vi "HAPS_MCU_Element_CMD.vi"(5 "set_ele":T3, 7 "HAPS_MCU_ELE_Func.":T2, 8 "error in":errorcluster, 11 "Function":T1={"Tx/Rx"=enum."Rx", "Enable?"=enum."On", "Source"=enum."MCU"}) -> (0 "error out":errorcluster, 3 "Data":string)   [LabVIEW 2023, in "HAPS.lvlib"]
uses:
  HAPS.lvlib
  HAPS_MCU_ELE_Func.ctl
  set_ele.ctl
  MCU_Function.ctl
panel:
  out "Time(ms)":dbl
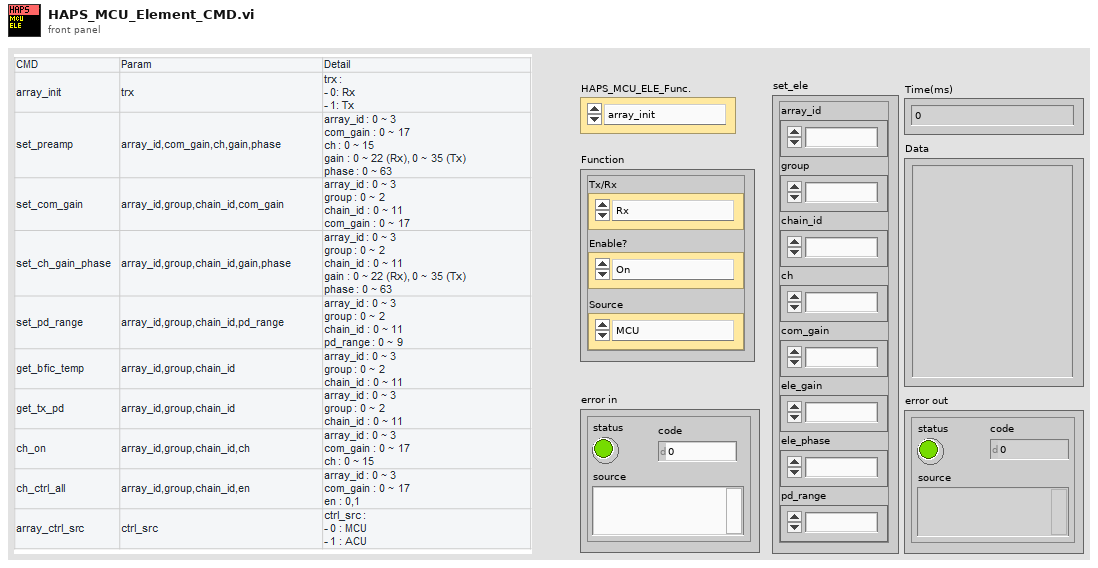
[diagram p1: front panel]
types:
  T1 = typedef "HAPS.lvlib/MCU_Function.ctl" = cluster{"Tx/Rx":enum16{"Rx", "Tx"}, "Enable?":enum16{"OFF", "On"}, "Source":enum16{"MCU", "ACU"}}
  T2 = typedef "HAPS.lvlib/HAPS_MCU_ELE_Func.ctl" = enum16{"array_init", "set_com_gain", "set_ch_gain_phase", "set_pd_range", "get_preamp_temp", "get_bfic_temp", "get_tx_pd", "ch_on", "ch_on_2", "ch_ctrl_all", "array_ctrl_src"}
  T3 = typedef "HAPS.lvlib/set_ele.ctl" = cluster{"ch":i32, "chain_id":i32, "group":i32, "array_id":i32, "ele_phase":i32, "ele_gain":i32, "com_gain":i32, "pd_range":i32}
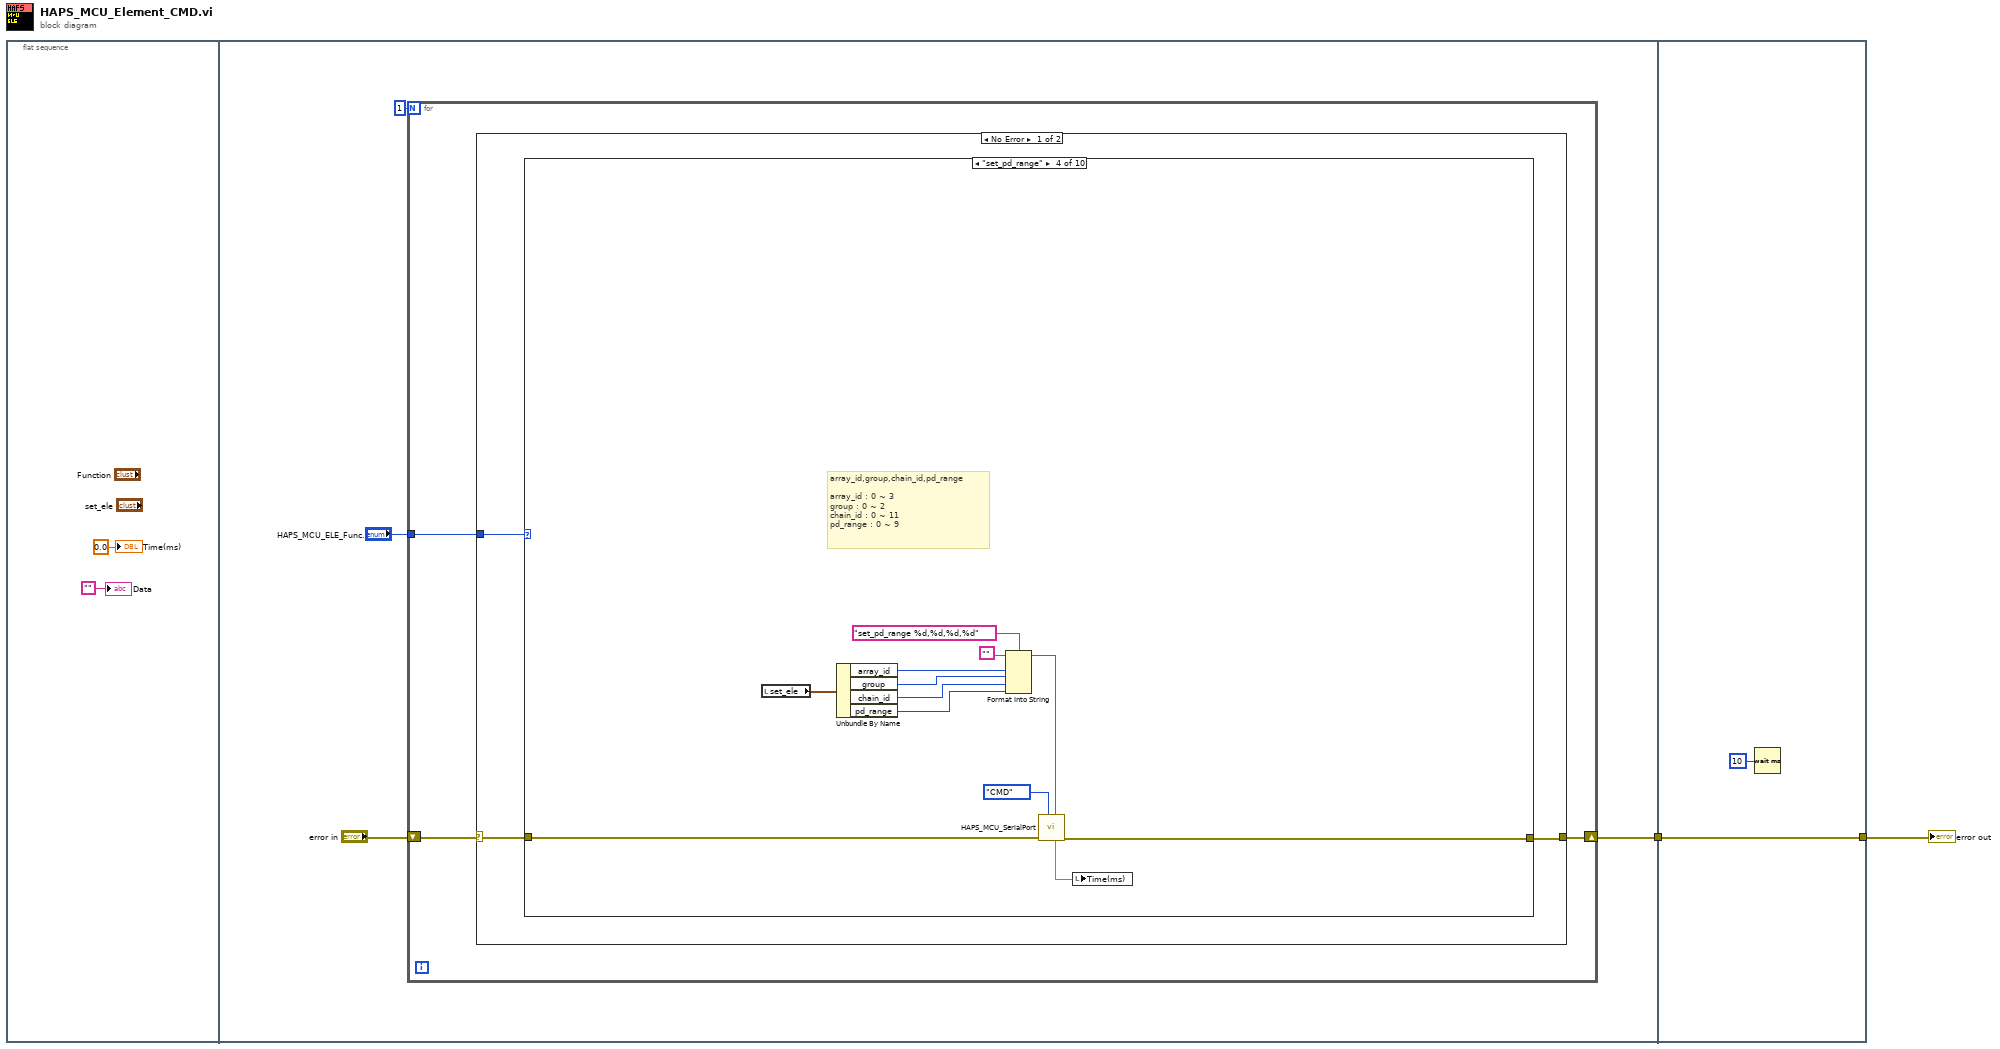
[diagram p0: block diagram]
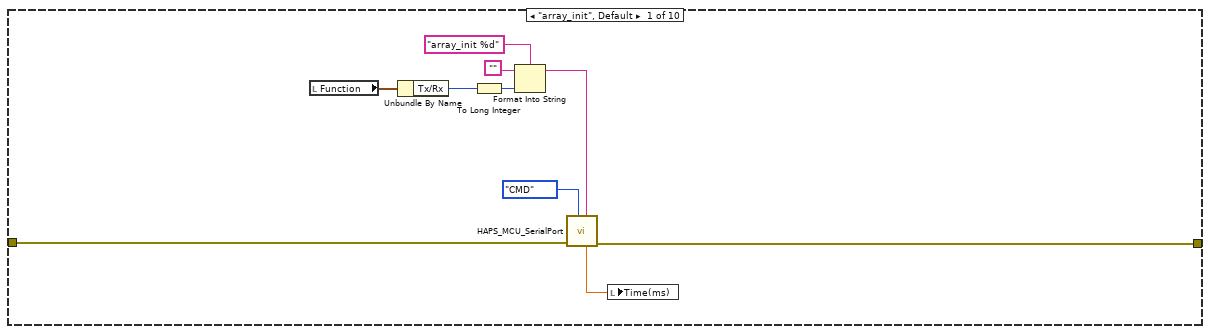
[diagram p2: hidden frame]
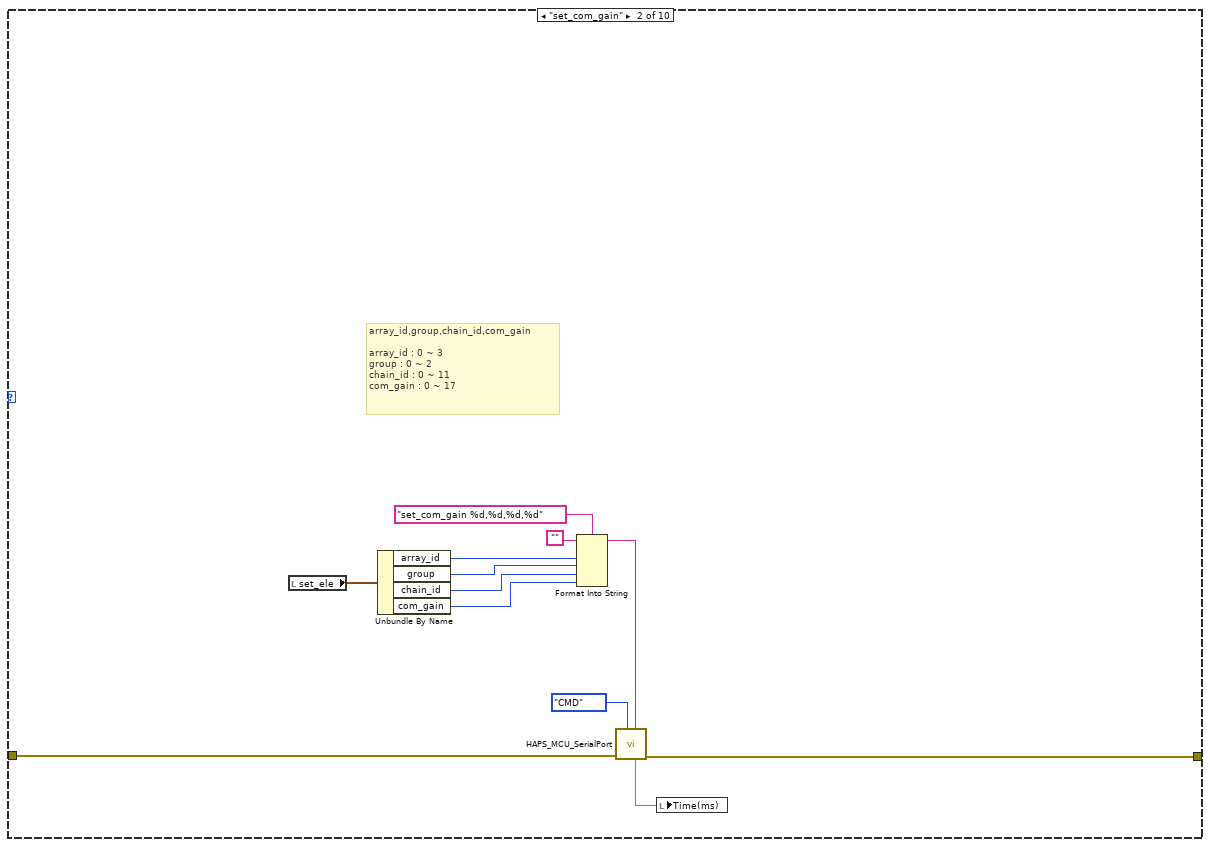
[diagram p3: hidden frame]
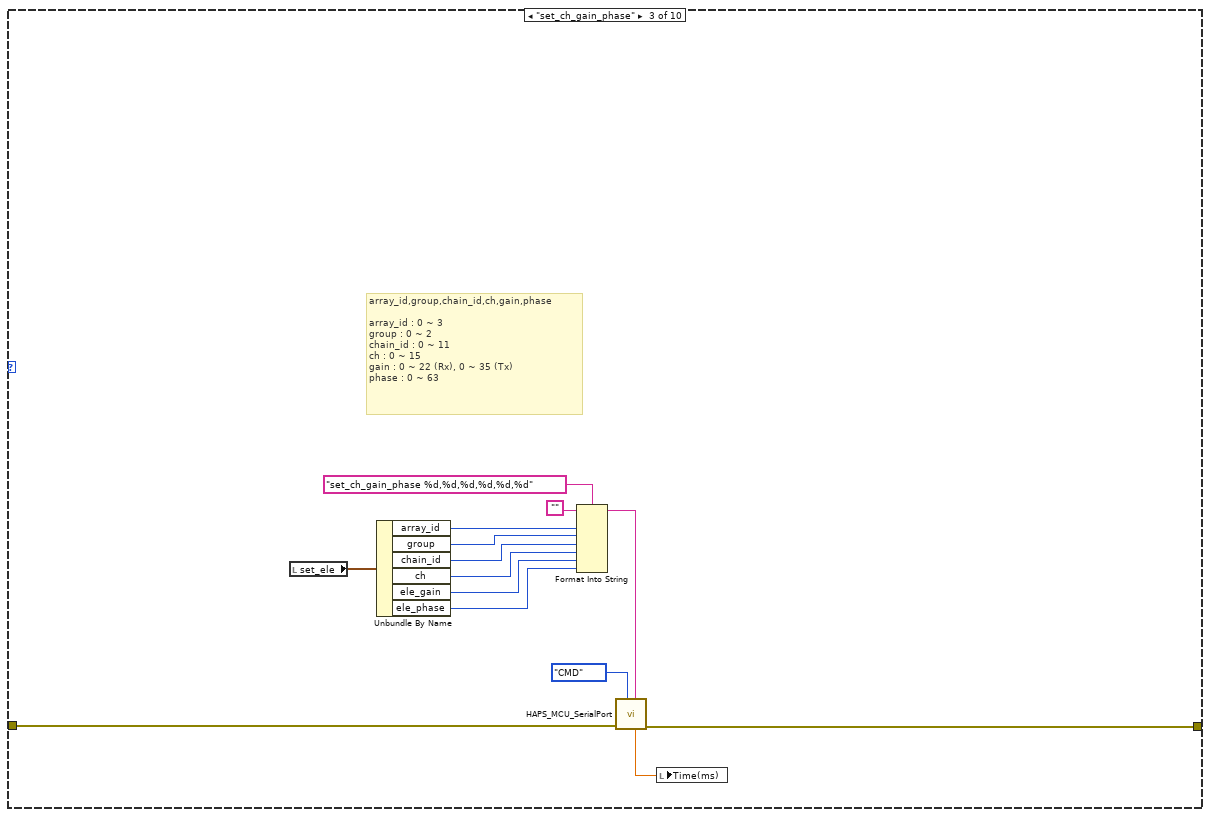
[diagram p4: hidden frame]
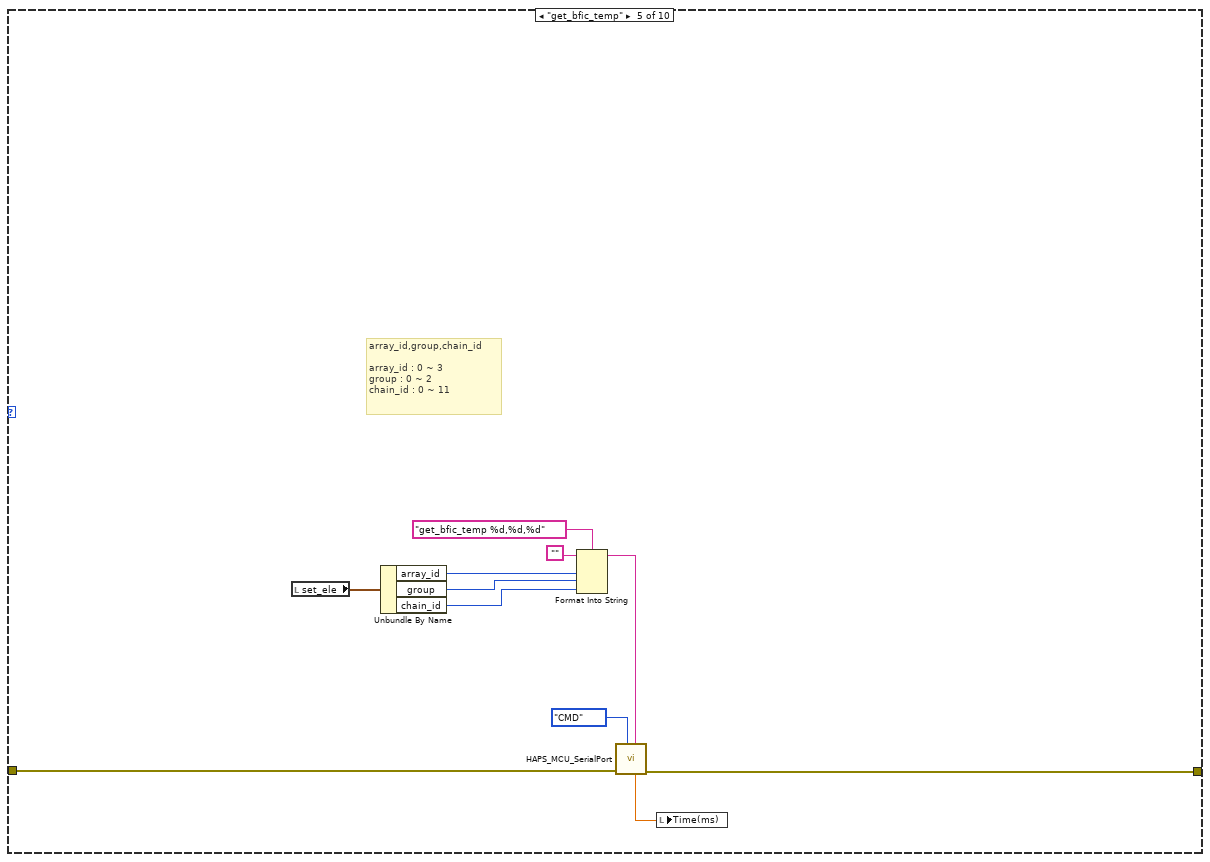
[diagram p5: hidden frame]
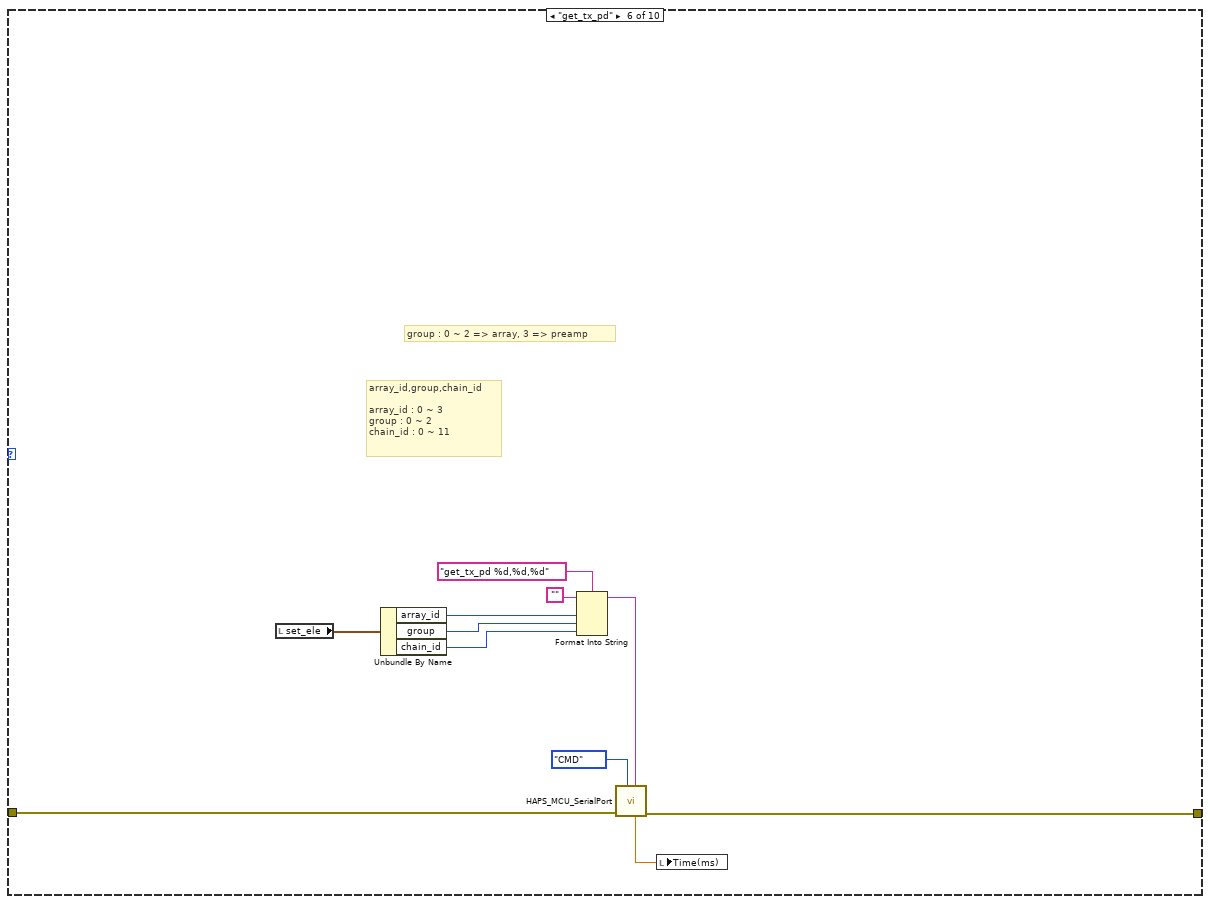
[diagram p6: hidden frame]
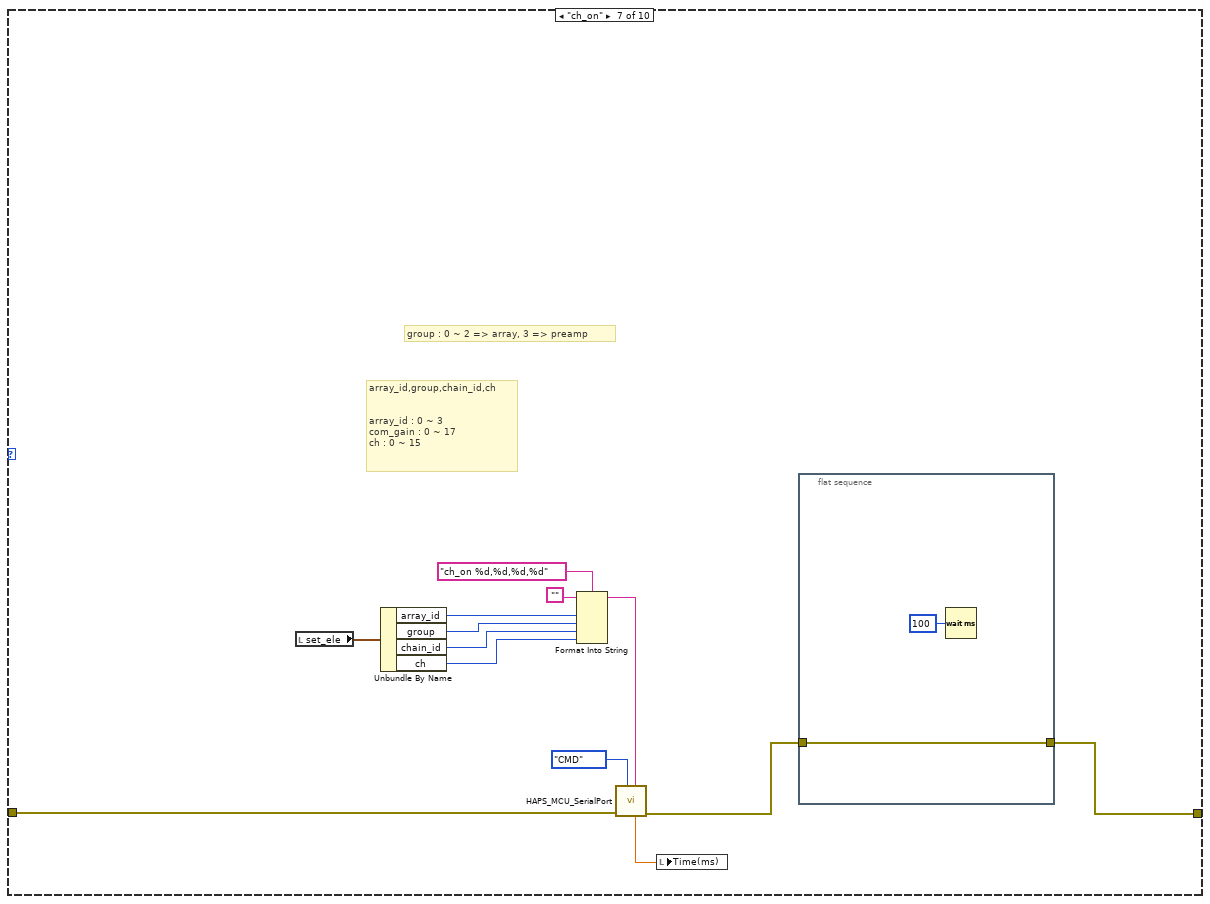
[diagram p7: hidden frame]
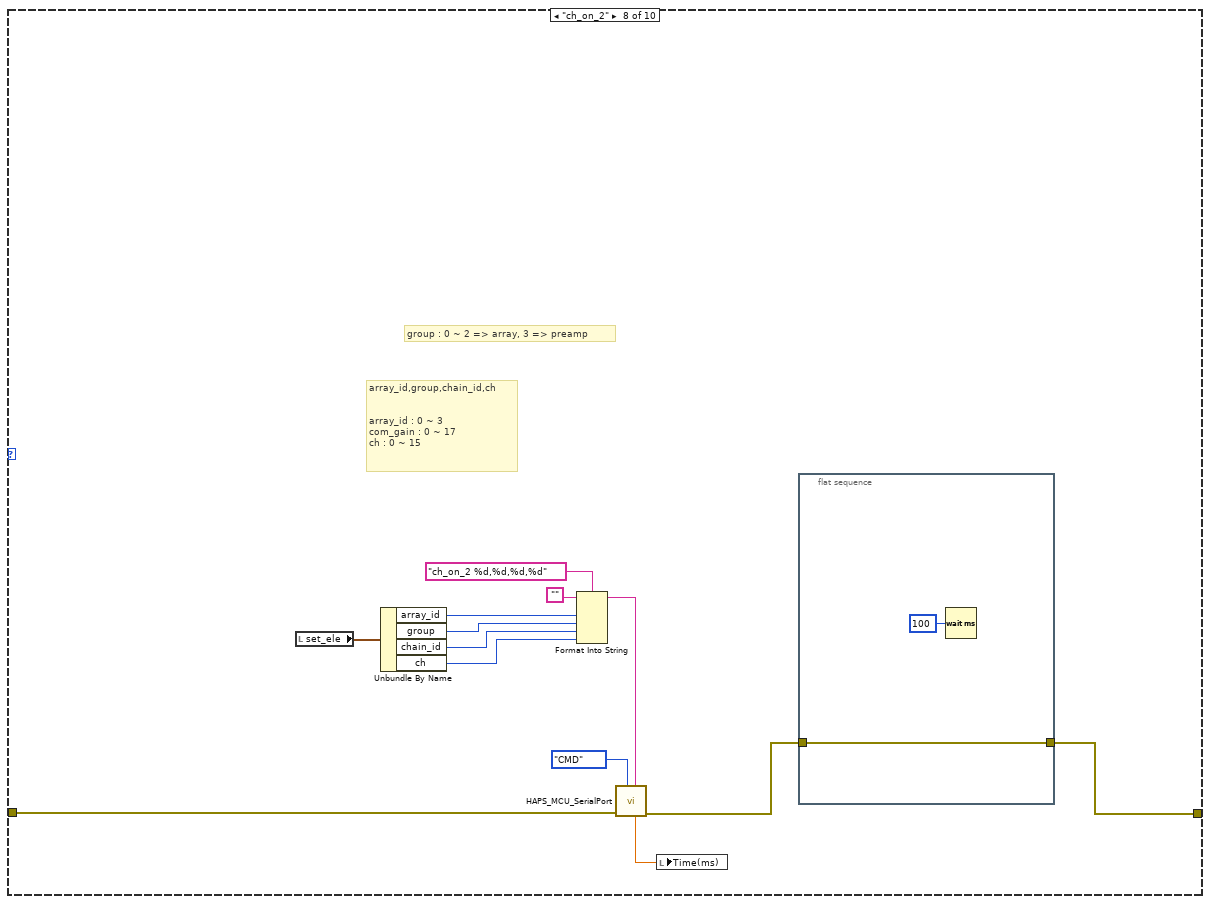
[diagram p8: hidden frame]
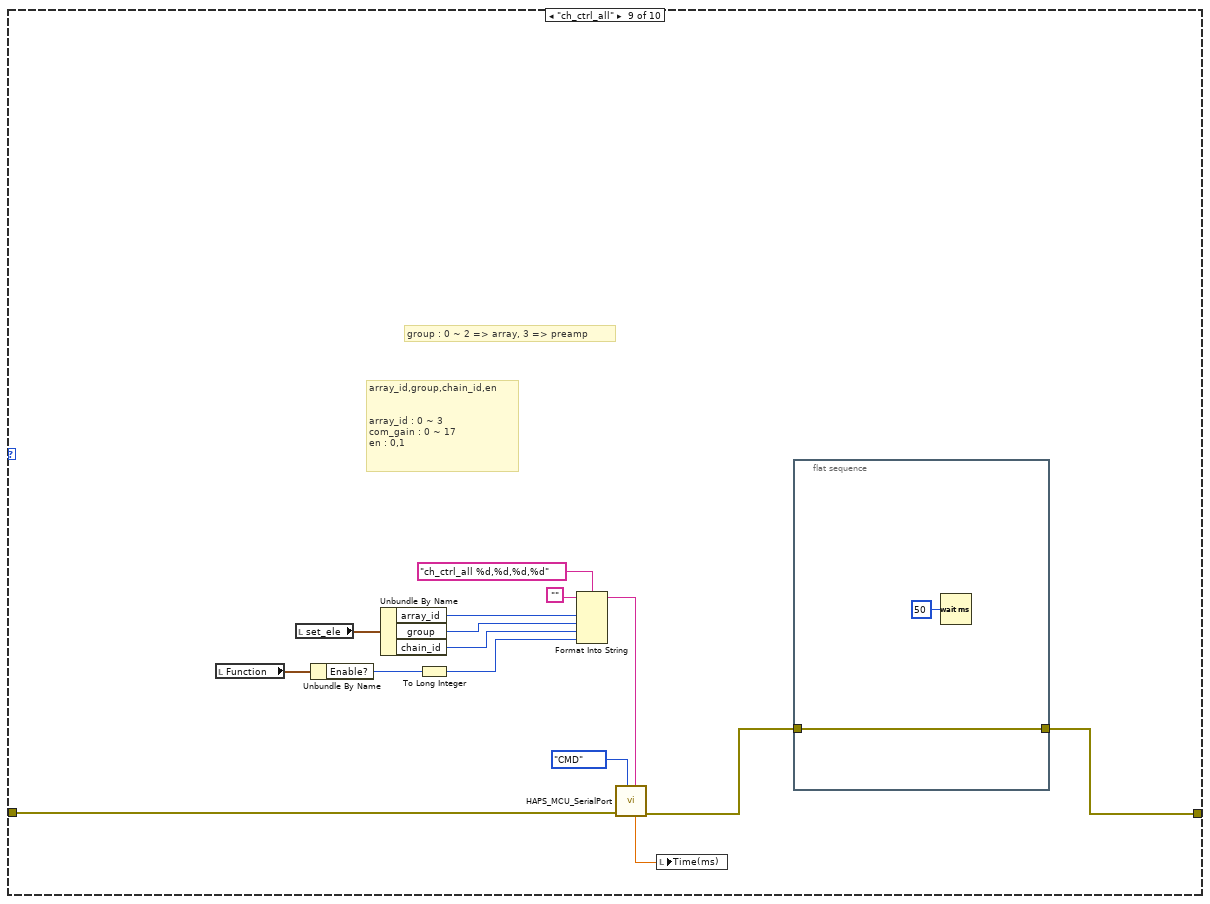
[diagram p9: hidden frame]
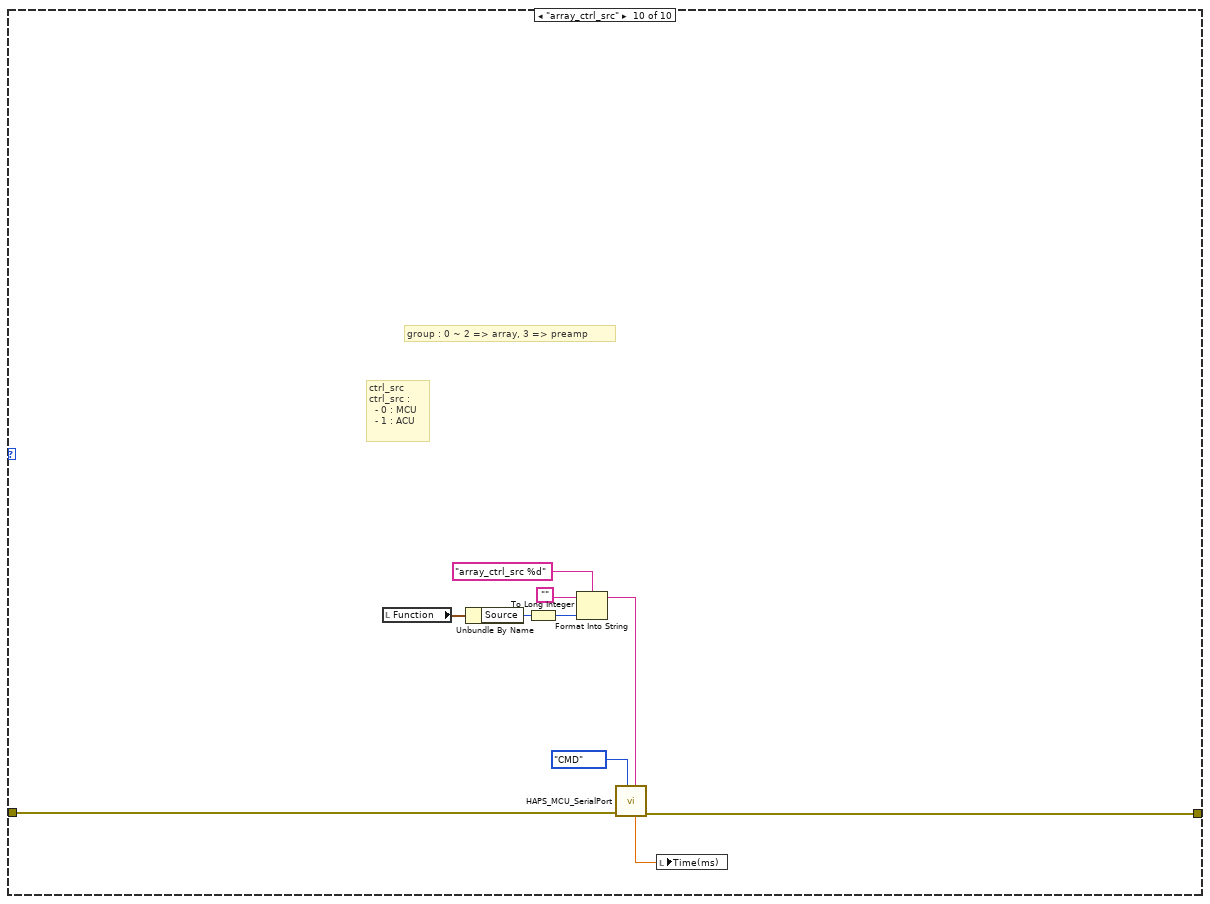
[diagram p10: hidden frame]
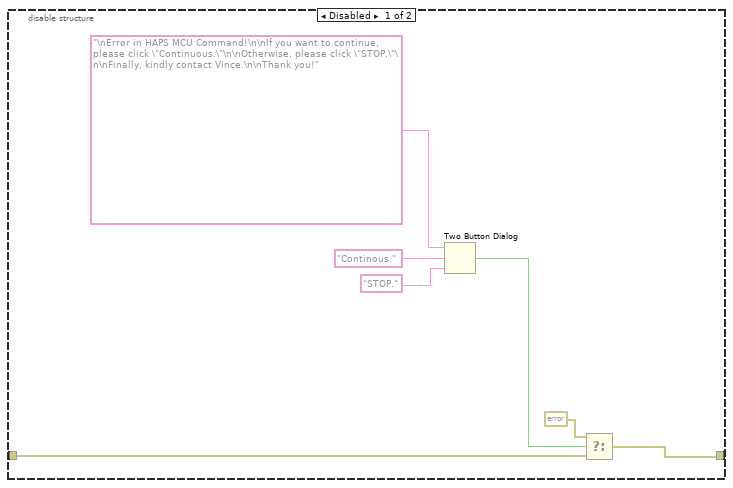
[diagram p12: hidden frame]
diagram:
  n1 = flat-sequence {
    tunnel: [w5] -> w1
    tunnel: [w153] -> w2
    tunnel: w1 -> [w153]
    frame #0 {
      "Time(ms)" <- 0.0 ("Time(ms)")
      "Data" <- ""
    }
    frame #1 {
      n2 = for {
        N: 1 -> [_]
        tunnel: "HAPS_MCU_ELE_Func." -> [w9]
        shift-right: [w11] -> w5
        shift-left: "error in" -> [w10]
        n3 = case shown="No Error" w10 {
          selector: w10 -> [w14 w143]
          tunnel: [w12 w142] -> w11
          tunnel: w9 -> [w13 _]
          frame No Error {
            n4 = case shown="\"set_pd_range\"" w13 {
              tunnel: w14 -> [w24 w36 w50 w62 w73 w84 w97 w112 w129 w141]
              tunnel: [w23 w35 w37 w61 w72 w83 w85 w100 w115 w140] -> w12
              frame "array_init", Default {
                n5 = local read "Function"() -> (w18:T1)
                n6 = Unbundle By Name(w18) -> ("Tx/Rx"=w15:enum16{"Rx", "Tx"})
                n7 = To Long Integer(number=w15) -> (32bit integer=w17:i32)
                n8 = Format Into String(format string="array_init %d" ("Command"), initial string="", w17) -> (resulting string=w16:string)  [unwired: 1 in, 1 out]
                n9 = call "HAPS_MCU_SerialPort.vi"("Command"=w16, "HAPS_SerialPort_Func"=enum16{"Init", "Close", "CMD"}."CMD" ("HAPS_SerialPort"), "error in"=w24) -> ("error out"=w23:errorcluster, "Time(ms)"=w22:dbl)  [unwired: 6 in, 1 out]
                n10 = local write "Time(ms)"(w22) -> ()
              }
              frame "set_com_gain" {
                # "array_id,group,chain_id,com_gain\n\narray_id : 0 ~ 3\ngroup : 0 ~ 2\nchain_id : 0 ~ 11\ncom_gain : 0 ~ 17"
                n11 = local read "set_ele"() -> (w25:T3)
                n12 = Unbundle By Name(w25) -> ("array_id"=w29:i32, "group"=w28:i32, "chain_id"=w27:i32, "com_gain"=w26:i32)
                n13 = Format Into String(format string="set_com_gain %d,%d,%d,%d" ("Command"), initial string="", w29, w28, w27, w26) -> (resulting string=w30:string)  [unwired: 1 in, 1 out]
                n14 = call "HAPS_MCU_SerialPort.vi"("Command"=w30, "HAPS_SerialPort_Func"=enum16{"Init", "Close", "CMD"}."CMD" ("HAPS_SerialPort"), "error in"=w36) -> ("error out"=w35:errorcluster, "Time(ms)"=w34:dbl)  [unwired: 6 in, 1 out]
                n15 = local write "Time(ms)"(w34) -> ()
              }
              frame "set_ch_gain_phase" {
                # "array_id,group,chain_id,ch,gain,phase\n\narray_id : 0 ~ 3\ngroup : 0 ~ 2\nchain_id : 0 ~ 11\nch : 0 ~ 15\ngain : 0 ~ 22 (Rx), 0 ~ 35 (Tx)\nphase : 0 ~ 63"
                n16 = local read "set_ele"() -> (w40:T3)
                n17 = Unbundle By Name(w40) -> ("array_id"=w44:i32, "group"=w43:i32, "chain_id"=w42:i32, "ch"=w41:i32, "ele_gain"=w39:i32, "ele_phase"=w38:i32)
                n18 = Format Into String(format string="set_ch_gain_phase %d,%d,%d,%d,%d,%d" ("Command"), initial string="", w44, w43, w42, w41, w39, w38) -> (resulting string=w45:string)  [unwired: 1 in, 1 out]
                n19 = call "HAPS_MCU_SerialPort.vi"("Command"=w45, "HAPS_SerialPort_Func"=enum16{"Init", "Close", "CMD"}."CMD" ("HAPS_SerialPort"), "error in"=w50) -> ("error out"=w37:errorcluster, "Time(ms)"=w49:dbl)  [unwired: 6 in, 1 out]
                n20 = local write "Time(ms)"(w49) -> ()
              }
              frame "set_pd_range" {
                # "array_id,group,chain_id,pd_range\n\narray_id : 0 ~ 3\ngroup : 0 ~ 2\nchain_id : 0 ~ 11\npd_range : 0 ~ 9"
                n21 = local read "set_ele"() -> (w51:T3)
                n22 = Unbundle By Name(w51) -> ("array_id"=w55:i32, "group"=w54:i32, "chain_id"=w53:i32, "pd_range"=w52:i32)
                n23 = Format Into String(format string="set_pd_range %d,%d,%d,%d" ("Command"), initial string="", w55, w54, w53, w52) -> (resulting string=w56:string)  [unwired: 1 in, 1 out]
                n24 = call "HAPS_MCU_SerialPort.vi"("Command"=w56, "HAPS_SerialPort_Func"=enum16{"Init", "Close", "CMD"}."CMD" ("HAPS_SerialPort"), "error in"=w62) -> ("error out"=w61:errorcluster, "Time(ms)"=w60:dbl)  [unwired: 6 in, 1 out]
                n25 = local write "Time(ms)"(w60) -> ()
              }
              frame "get_bfic_temp" {
                # "array_id,group,chain_id\n\narray_id : 0 ~ 3\ngroup : 0 ~ 2\nchain_id : 0 ~ 11"
                n26 = local read "set_ele"() -> (w63:T3)
                n27 = Unbundle By Name(w63) -> ("array_id"=w66:i32, "group"=w65:i32, "chain_id"=w64:i32)
                n28 = Format Into String(format string="get_bfic_temp %d,%d,%d" ("Command"), initial string="", w66, w65, w64) -> (resulting string=w67:string)  [unwired: 1 in, 1 out]
                n29 = call "HAPS_MCU_SerialPort.vi"("Command"=w67, "HAPS_SerialPort_Func"=enum16{"Init", "Close", "CMD"}."CMD" ("HAPS_SerialPort"), "error in"=w73) -> ("error out"=w72:errorcluster, "Time(ms)"=w71:dbl)  [unwired: 6 in, 1 out]
                n30 = local write "Time(ms)"(w71) -> ()
              }
              frame "get_tx_pd" {
                # "group : 0 ~ 2 => array, 3 => preamp"
                # "array_id,group,chain_id\n\narray_id : 0 ~ 3\ngroup : 0 ~ 2\nchain_id : 0 ~ 11"
                n31 = local read "set_ele"() -> (w76:T3)
                n32 = Unbundle By Name(w76) -> ("array_id"=w77:i32, "group"=w75:i32, "chain_id"=w74:i32)
                n33 = Format Into String(format string="get_tx_pd %d,%d,%d" ("Command"), initial string="", w77, w75, w74) -> (resulting string=w78:string)  [unwired: 1 in, 1 out]
                n34 = call "HAPS_MCU_SerialPort.vi"("Command"=w78, "HAPS_SerialPort_Func"=enum16{"Init", "Close", "CMD"}."CMD" ("HAPS_SerialPort"), "error in"=w84) -> ("error out"=w83:errorcluster, "Time(ms)"=w82:dbl)  [unwired: 6 in, 1 out]
                n35 = local write "Time(ms)"(w82) -> ()
              }
              frame "ch_on" {
                # "group : 0 ~ 2 => array, 3 => preamp"
                # "array_id,group,chain_id,ch\n\n\narray_id : 0 ~ 3\ncom_gain : 0 ~ 17\nch : 0 ~ 15"
                n36 = local read "set_ele"() -> (w90:T3)
                n37 = Unbundle By Name(w90) -> ("array_id"=w91:i32, "group"=w89:i32, "chain_id"=w88:i32, "ch"=w87:i32)
                n38 = Format Into String(format string="ch_on %d,%d,%d,%d" ("Command"), initial string="", w91, w89, w88, w87) -> (resulting string=w92:string)  [unwired: 1 in, 1 out]
                n39 = call "HAPS_MCU_SerialPort.vi"("Command"=w92, "HAPS_SerialPort_Func"=enum16{"Init", "Close", "CMD"}."CMD" ("HAPS_SerialPort"), "error in"=w97) -> ("error out"=w86:errorcluster, "Time(ms)"=w96:dbl)  [unwired: 6 in, 1 out]
                n40 = local write "Time(ms)"(w96) -> ()
                n41 = flat-sequence {
                  tunnel: w86 -> [w98]
                  tunnel: [w98] -> w85
                  frame #0 {
                    n42 = Wait (ms)(milliseconds to wait=u32 100) -> ()  [unwired: 1 out]
                  }
                }
              }
              frame "ch_on_2" {
                # "group : 0 ~ 2 => array, 3 => preamp"
                # "array_id,group,chain_id,ch\n\n\narray_id : 0 ~ 3\ncom_gain : 0 ~ 17\nch : 0 ~ 15"
                n43 = local read "set_ele"() -> (w105:T3)
                n44 = Unbundle By Name(w105) -> ("array_id"=w106:i32, "group"=w104:i32, "chain_id"=w103:i32, "ch"=w102:i32)
                n45 = Format Into String(format string="ch_on_2 %d,%d,%d,%d" ("Command"), initial string="", w106, w104, w103, w102) -> (resulting string=w107:string)  [unwired: 1 in, 1 out]
                n46 = call "HAPS_MCU_SerialPort.vi"("Command"=w107, "HAPS_SerialPort_Func"=enum16{"Init", "Close", "CMD"}."CMD" ("HAPS_SerialPort"), "error in"=w112) -> ("error out"=w101:errorcluster, "Time(ms)"=w111:dbl)  [unwired: 6 in, 1 out]
                n47 = local write "Time(ms)"(w111) -> ()
                n48 = flat-sequence {
                  tunnel: w101 -> [w113]
                  tunnel: [w113] -> w100
                  frame #0 {
                    n49 = Wait (ms)(milliseconds to wait=u32 100) -> ()  [unwired: 1 out]
                  }
                }
              }
              frame "ch_ctrl_all" {
                # "group : 0 ~ 2 => array, 3 => preamp"
                # "array_id,group,chain_id,en\n\n\narray_id : 0 ~ 3\ncom_gain : 0 ~ 17\nen : 0,1"
                n50 = local read "Function"() -> (w119:T1)
                n51 = local read "set_ele"() -> (w122:T3)
                n52 = Unbundle By Name(w119) -> ("Enable?"=w117:enum16{"OFF", "On"})
                n53 = Unbundle By Name(w122) -> ("array_id"=w123:i32, "group"=w121:i32, "chain_id"=w120:i32)
                n54 = To Long Integer(number=w117) -> (32bit integer=w118:i32)
                n55 = Format Into String(format string="ch_ctrl_all %d,%d,%d,%d" ("Command"), initial string="", w123, w121, w120, w118) -> (resulting string=w124:string)  [unwired: 1 in, 1 out]
                n56 = call "HAPS_MCU_SerialPort.vi"("Command"=w124, "HAPS_SerialPort_Func"=enum16{"Init", "Close", "CMD"}."CMD" ("HAPS_SerialPort"), "error in"=w129) -> ("error out"=w116:errorcluster, "Time(ms)"=w128:dbl)  [unwired: 6 in, 1 out]
                n57 = local write "Time(ms)"(w128) -> ()
                n58 = flat-sequence {
                  tunnel: w116 -> [w130]
                  tunnel: [w130] -> w115
                  frame #0 {
                    n59 = Wait (ms)(milliseconds to wait=u32 50) -> ()  [unwired: 1 out]
                  }
                }
              }
              frame "array_ctrl_src" {
                # "group : 0 ~ 2 => array, 3 => preamp"
                # "ctrl_src\nctrl_src : \n  - 0 : MCU\n  - 1 : ACU"
                n60 = local read "Function"() -> (w134:T1)
                n61 = Unbundle By Name(w134) -> ("Source"=w132:enum16{"MCU", "ACU"})
                n62 = To Long Integer(number=w132) -> (32bit integer=w133:i32)
                n63 = Format Into String(format string="array_ctrl_src %d" ("Command"), initial string="", w133) -> (resulting string=w135:string)  [unwired: 1 in, 1 out]
                n64 = call "HAPS_MCU_SerialPort.vi"("Command"=w135, "HAPS_SerialPort_Func"=enum16{"Init", "Close", "CMD"}."CMD" ("HAPS_SerialPort"), "error in"=w141) -> ("error out"=w140:errorcluster, "Time(ms)"=w139:dbl)  [unwired: 6 in, 1 out]
                n65 = local write "Time(ms)"(w139) -> ()
              }
            }
          }
          frame Error {
            n66 = disable-structure shown="Enabled" {
              disable-tunnel: w143 -> [w146 w151]
              disable-tunnel: [w144 w151] -> w142
              frame Disabled {
                n67 = Two Button Dialog(message="\nError in HAPS MCU Command!\n\nIf you want to continue, please click \"Continuous.\"\n\nOtherwise, please click \"STOP.\"\n\nFinally, kindly contact Vince.\n\nThank you!", 1:"STOP." ("F button name (\"Cancel\")"), 2:"Continous." ("T button name (\"OK\")")) -> (T button?=w147:bool)
                n68 = Select(t=errorcluster {"status"=FALSE, "code"=0, "source"=""}, s=w147, f=w146) -> (s? t:f=w144:errorcluster)
              }
              frame Enabled {
              }
            }
          }
        }
      }
    }
    frame #2 {
      n69 = Wait (ms)(milliseconds to wait=u32 10) -> ()  [unwired: 1 out]
    }
  }
  "error out" <- w2
